vi "MPXV4006G Calibration.vi"(2 "error in (no error)":errorcluster, 3 "Sensor Voltage":dbl) -> (0 "error out":errorcluster, 1 "Pressure":dbl)   [LabVIEW 2017]
uses:
  <vilib>/gmath/NI_Gmath.lvlib
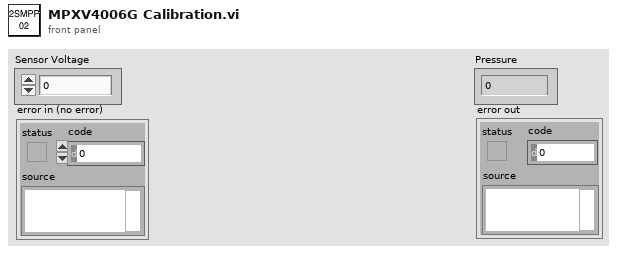
[diagram p1: front panel]
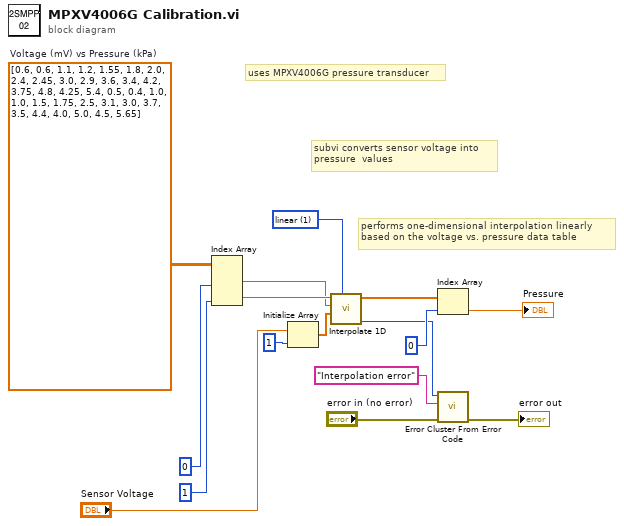
[diagram p0: block diagram]
diagram:
  w8 = 1 items=["nearest", "linear", "spline", "cubic Hermite", "Lagrange"] ("method")
  w16 = dbl[][] [[0.6, 0.6], [1.1, 1.2], [1.55, 1.8], [2.0, 2.4], [2.45, 3.0], [2.9, 3.6], [3.4, 4.2], [3.75, 4.8], [4.25, 5.4], [0.5, 0.4], [1.0, 1.0], [1.5, 1.75], [2.5, 3.1], [3.0, 3.7], [3.5, 4.4], [4.0, 5.0], [4.5, 5.65]]  # Voltage (mV) vs Pressure (kPa)
  # "uses MPXV4006G pressure transducer"
  # "performs one-dimensional interpolation linearly\nbased on the voltage vs. pressure data table"
  # "subvi converts sensor voltage into \npressure  values"
  n1 = Index Array "Index Array"(array=w16, index (col) #1=0 ("disabled index (col)"), index (col) #2=1 ("index (col)")) -> (element #1=w12:dbl[], element #2=w13:dbl[])  [unwired: 2 in]
  n2 = Initialize Array "Initialize Array"("Sensor Voltage", 1 ("dimension size")) -> (w10:dbl[])
  n3 = call <vilib>:"Interpolate 1D.vi"("method"=w8, "xi"=w10, "X"=w12, "Y"=w13) -> ("error"=w4:i32, "yi"=w7:dbl[])  [unwired: 5 in, 1 out]
  n4 = Index Array "Index Array"(array=w7, index=0) -> (element=→"Pressure":dbl)
  n5 = call <vilib>:"Error Cluster From Error Code.vi"("error in (no error)"="error in (no error)", "error message (\"\")"="Interpolation error" ("error message (\"\")"), "error code (0)"=w4) -> ("error out"=→"error out":errorcluster)  [unwired: 6 in]
